vi "Convert 2D to Waveform Array LV2012 NIVerified.vi"(9 "Data":dbl[][](array[numeric]), 10 "dt":dbl, 11 "t0":timestamp) -> (2 "Waveform Array Out":waveform(dbl)[](array[waveform]), 3 "New t0":timestamp)   [LabVIEW 2020]
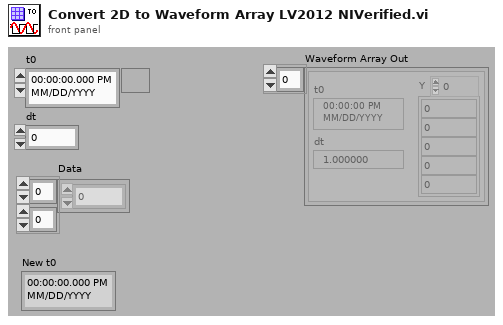
[diagram p1: front panel]
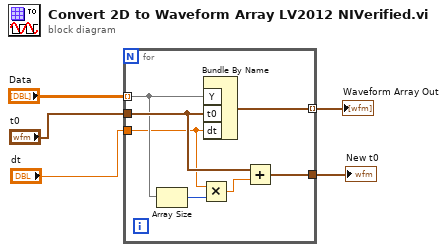
[diagram p0: block diagram]
diagram:
  n1 = for {
    tunnel: "Data" -> [w10] mode=indexing
    tunnel: [w12] -> w4 mode=indexing
    tunnel: "t0" -> [w11]
    tunnel: "dt" -> [w8]
    tunnel: [w6] -> w1
    n2 = Array Size(array=w10) -> (size(s)=w9:i32)
    n3 = Multiply(x=w8, y=w9) -> (x*y=w7:dbl)
    n4 = Bundle By Name("Y"=w10, "t0"=w11, "dt"=w8) -> (w12:waveform(dbl))  [unwired: 1 in]
    n5 = Add(x=w11, y=w7) -> (x+y=w6:timestamp)
  }
  "Waveform Array Out" <- w4
  "New t0" <- w1
